vi "isItRunning.vi"(8 "error in (no error)":errorcluster, 11 "CameraControlViewer in":refnum<class "CameraControlViewer.lvclass">) -> (0 "error out":errorcluster, 2 "running?":bool, 3 "CameraControlViewer out":refnum<class "CameraControlViewer.lvclass">)   [LabVIEW 2011, in "Views.lvlib" / "Camera.lvlib" / "CameraControlViewer.lvclass"]
uses:
  CameraControlViewer.lvclass
  CameraControlViewer.lvclass/CameraControlViewer.ctl
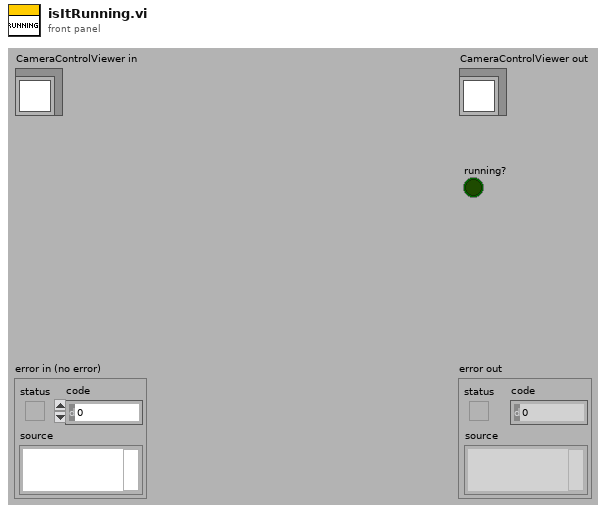
[diagram p1: front panel]
types:
  T1 = enum32{"Bad", "Idle", "Run top level", "Running"}
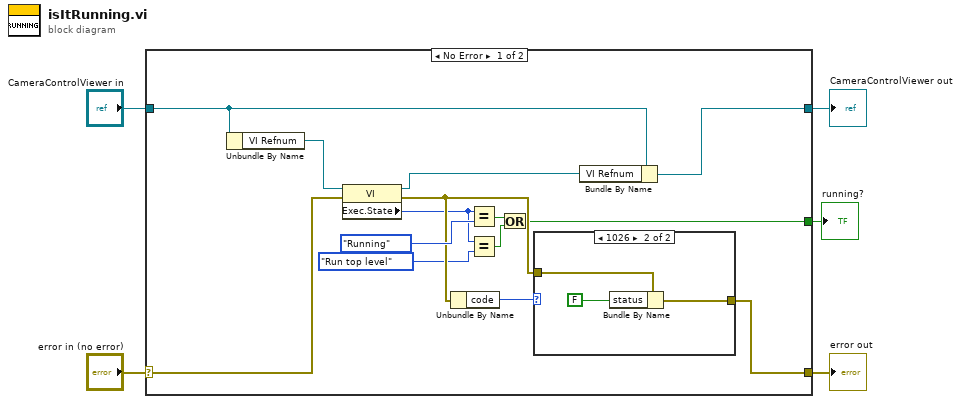
[diagram p0: block diagram]
diagram:
  n1 = case shown="No Error" "error in (no error)" {
    selector: "error in (no error)" -> [w10 w25]
    tunnel: [w7 w25] -> w4
    tunnel: [w8 w24] -> w2
    tunnel: "CameraControlViewer in" -> [w9 w24]
    tunnel: [w6 _] -> w1
    frame No Error {
      n2 = Unbundle By Name(w9) -> ("VI Refnum"=w11:refnum<vi>)
      n3 = property class="VI"(reference=w11, error in=w10) -> (reference out=w18:refnum<vi>, error out=w16:errorcluster, "Exec.State"=w15:T1)
      n4 = Unbundle By Name(w16) -> ("code"=w17:i32)
      n5 = Equal?(x=w15, y=T1."Running" ("Execution:State")) -> (x = y?=w13:bool)
      n6 = Equal?(x=w15, y=T1."Run top level" ("Execution:State")) -> (x = y?=w12:bool)
      n7 = Or(x=w13, y=w12) -> (x .or. y?=w6:bool)
      n8 = case shown="1026" w17 {
        tunnel: w16 -> [w20 w23]
        tunnel: [w20 w22] -> w7
        frame 0, Default {
        }
        frame 1026 {
          n9 = Bundle By Name(cluster=w23, "status"=FALSE) -> (w22:errorcluster)
        }
      }
      n10 = Bundle By Name(cluster=w9, "VI Refnum"=w18) -> (w8:refnum<class "CameraControlViewer.lvclass">)
    }
    frame Error {
    }
  }
  "error out" <- w4
  "CameraControlViewer out" <- w2
  "running?" <- w1
